vi "Scrip_execution_v02.vi"() -> (3 "添加的数组":string[](array[string]))   [LabVIEW 2024]
panel:
  out "添加的数组 2":bool[](array[boolean])
  out "遍历vi名称":string[](array[string])
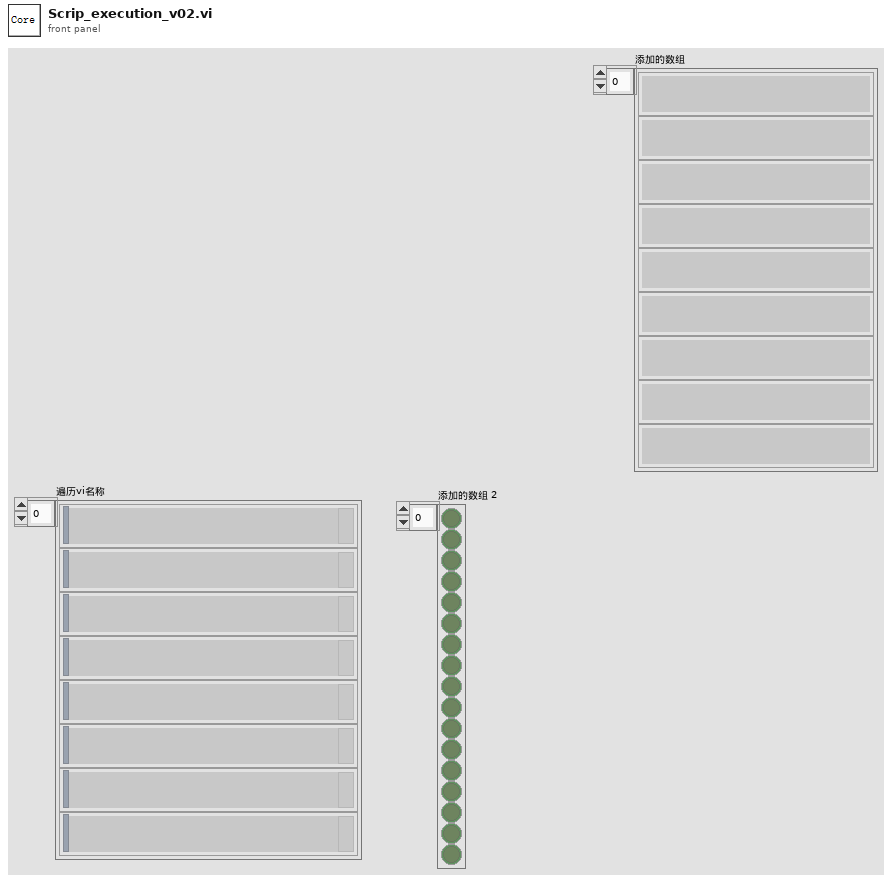
[diagram p1: front panel]
types:
  T1 = cluster{"元素":string, "元素 2":string, "元素 3":string, "元素 4":string, "元素 5":string, "元素 6":string, "元素 7":string, "元素 8":string, "元素 9":string, "元素 10":string, "元素 11":string, "元素 12":string, "元素 13":string, "元素 14":string, "元素 15":string}[]
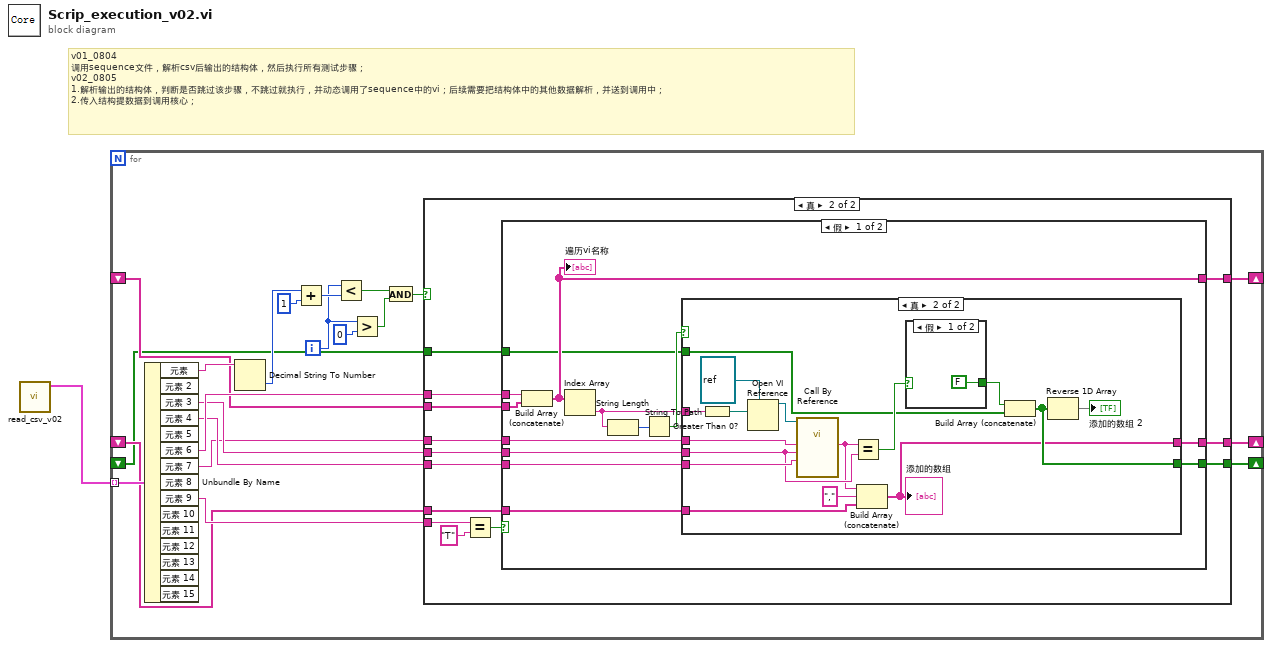
[diagram p0: block diagram]
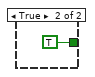
[diagram p4: hidden frame]
diagram:
  # "v01_0804\n调用sequence文件，解析csv后输出的结构体，然后执行所有测试步骤；\nv02_0805\n1.解析输出的结构体，判断是否跳过该步骤，不跳过就执行，并动态调用了sequence中的vi；后续需要把结构体中的其他数据解析，并送到调用中；\n2.传入结构提数据到调用核心；"
  n1 = call "read_csv_v02.vi"() -> ("目标结构体数组"=w1:T1)  [unwired: 10 in, 1 out]
  n2 = for {
    tunnel: w1 -> [w22] mode=indexing
    shift-right: [w10] -> _
    shift-left: _ -> [w9]
    shift-right: [w8] -> _
    shift-left: _ -> [w7]
    shift-right: [w5] -> _
    shift-left: _ -> [w4]
    i -> [w16]
    n3 = Unbundle By Name(w22) -> ("元素"=w20:string, "元素 3"=w3:string, "元素 4"=w6:string, "元素 6"=w11:string, "元素 7"=w2:string, "元素 9"=w21:string)  [unwired: 9 out]
    n4 = Decimal String To Number(string=w20) -> (number=w19:i32)  [unwired: 2 in, 1 out]
    n5 = Add(x=w19, y=1) -> (x+y=w17:i32)
    n6 = Less?(x=w16, y=w17) -> (x < y?=w14:bool)
    n7 = Greater?(x=w16, y=0) -> (0:w13:bool)
    n8 = And(x=w14, y=w13) -> (x .and. y?=w12:bool)
    n9 = case shown="真" w12 {
      tunnel: w21 -> [_ w33]
      tunnel: w11 -> [_ w32]
      tunnel: [_ w31] -> w10
      tunnel: w9 -> [_ w30]
      tunnel: [_ w29] -> w8
      tunnel: w7 -> [_ w28]
      tunnel: w2 -> [_ w27]
      tunnel: w3 -> [_ w26]
      tunnel: w6 -> [_ w25]
      tunnel: [_ w24] -> w5
      tunnel: w4 -> [_ w23]
      frame False {
      }
      frame True {
        n10 = Equal?(x=w33, y="T") -> (x = y?=w34:bool)
        n11 = case shown="假" w34 {
          tunnel: w32 -> [w47 _]
          tunnel: [w46 _] -> w31
          tunnel: w30 -> [w48 _]
          tunnel: [w43 _] -> w29
          tunnel: w28 -> [w42 _]
          tunnel: w27 -> [w40 _]
          tunnel: w26 -> [w39 _]
          tunnel: w25 -> [w38 _]
          tunnel: [w37 _] -> w24
          tunnel: w23 -> [w36 _]
          frame False {
            n12 = Build Array (concatenate)(w47, w48) -> (w46:string[])
            "遍历vi名称" <- w46
            n13 = Index Array(array=w46) -> (element=w41:string)  [unwired: 1 in]
            n14 = String Length(string=w41) -> (length=w45:i32)
            n15 = Greater Than 0?(x=w45) -> (x > 0?=w44:bool)
            n16 = case shown="真" w44 {
              tunnel: w41 -> [_ w63]
              tunnel: [_ w51] -> w43
              tunnel: w42 -> [_ w50]
              tunnel: w40 -> [_ w62]
              tunnel: w39 -> [_ w58]
              tunnel: w38 -> [_ w59]
              tunnel: [_ w54] -> w37
              tunnel: w36 -> [_ w55]
              frame False {
              }
              frame True {
                n17 = String To Path(string=w63) -> (path=w64:path)
                n18 = Open VI Reference(type specifier VI Refnum (for type only)=refnum<vi> refnum ("类型说明符VI引用句柄（仅用于类型）"), vi path=w64) -> (vi reference=w60:refnum<vi>)  [unwired: 4 in, 1 out]
                n19 = call-by-ref "?"(reference=w60, "Low_Litmit"=w59, "High_Litmit"=w58, "SN"=w62) -> ("元素"=w52:string)  [unwired: 7 in, 4 out]
                n20 = Equal?(x=w52, y=w58) -> (x = y?=w57:bool)
                n21 = Build Array (concatenate)(w52, "," ("元素 4"), w50) -> (w51:string[])
                "添加的数组" <- w51
                n22 = case shown="假" w57 {
                  tunnel: [FALSE ("布尔") TRUE ("布尔")] -> w56
                  frame False {
                  }
                  frame True {
                  }
                }
                n23 = Build Array (concatenate)(w56, w55) -> (w54:bool[])
                n24 = Reverse 1D Array(array=w54) -> (reversed array=→"添加的数组 2":bool[])
              }
            }
          }
          frame True {
          }
        }
      }
    }
  }
